vi "max obrot jazda.vi"(9 "Z axis":i32, 10 "max obrót":i32) -> (3 "y":i32)   [LabVIEW 2015]
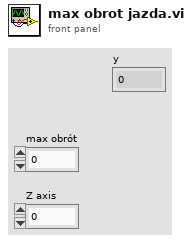
[diagram p1: front panel]
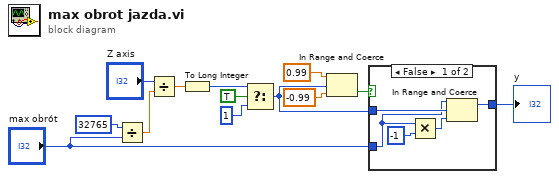
[diagram p0: block diagram]
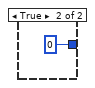
[diagram p2: hidden frame]
diagram:
  n1 = Divide(x=32765 ("y"), y="max obrót") -> (x/y=w10:dbl)
  n2 = Divide(x="Z axis", y=w10) -> (x/y=w8:dbl)
  n3 = To Long Integer(number=w8) -> (32bit integer=w7:i32)
  n4 = Select(t=w7, s=TRUE, f=1) -> (s? t:f=w4:i32)
  n5 = In Range and Coerce(upper limit=0.99 ("y"), x=w4, lower limit=-0.99 ("y")) -> (In Range?=w3:bool)  [unwired: 1 out]
  n6 = case shown="False" w3 {
    tunnel: [w18 0 ("y")] -> w12
    tunnel: w4 -> [w15 _]
    tunnel: "max obrót" -> [w14 _]
    frame False {
      n7 = Multiply(x=w14, y=-1) -> (x*y=w17:i32)
      n8 = In Range and Coerce(upper limit=w14, x=w15, lower limit=w17) -> (coerced(x)=w18:i32)  [unwired: 1 out]
    }
    frame True {
    }
  }
  "y" <- w12
